vi "Keep_Find.vi"(1 "x":string="flat", 2 "rawlist":string[][](array[string]), 3 "sequence":T1) -> (0 "index":i32)   [LabVIEW 2010]
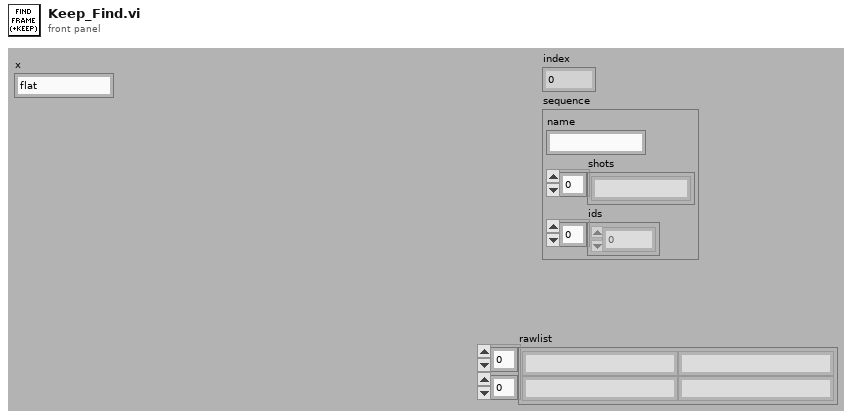
[diagram p1: front panel]
types:
  T1 = cluster{"name":string, "shots":string[], "ids":i32[]}
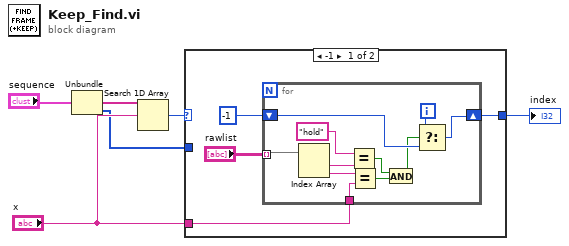
[diagram p0: block diagram]
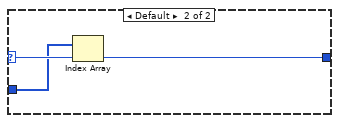
[diagram p2: hidden frame]
diagram:
  n1 = Unbundle("sequence") -> ("shots"=w5:string[], "ids"=w2:i32[])  [unwired: 1 out]
  n2 = Search 1D Array(1D array=w5, element="x") -> (index of element=w4:i32)  [unwired: 1 in]
  n3 = case shown="-1" w4 {
    selector: w4 -> [_ w24]
    tunnel: "x" -> [w8 _]
    tunnel: w2 -> [_ w23]
    tunnel: [w7 w22] -> w1
    frame -1 {
      n4 = for {
        tunnel: "rawlist" -> [w21] mode=indexing
        shift-right: [w12] -> w7
        shift-left: -1 -> [w13]
        tunnel: w8 -> [w17]
        i -> [w14]
        n5 = Index Array(array=w21) -> (element #1=w20:string, element #2=w19:string)  [unwired: 2 in]
        n6 = Equal?(x="hold", y=w20) -> (x = y?=w16:bool)
        n7 = Equal?(x=w19, y=w17) -> (x = y?=w15:bool)
        n8 = And(x=w16, y=w15) -> (x .and. y?=w11:bool)
        n9 = Select(t=w14, s=w11, f=w13) -> (s? t:f=w12:i32)
      }
    }
    frame Default {
      n10 = Index Array(array=w23, index=w24) -> (element=w22:i32)
    }
  }
  "index" <- w1
